vi "4. MassData in CSM.vi"() -> ()   [LabVIEW 2017]
doc: "## Using MassData in the CSM Framework (4. MassData in CSM.vi)\n\n### Overview\n\nDemonstrates how to use MassData within the CSM framework.\n\n### Introduction\n\nThis example uses a Producer/Consumer scenario to show how MassData operates within the CSM context.\n\nA non-CSM loop acts as the data producer, responsible for generating data, packing the data into a MassData argument, and sending the data via a synchronous message to the CSM module, which acts as the data consumer. This example demonstrates this process.\n\n### Steps\n\n- Step 1: Use `CSM - Config MassData Parameter Cache Size.vi` to set the cache size.\n- Step 2: Data producer loop. This loop is not a CSM module.\n - Step 2.1: Construct raw data, which in a real-world program comes from hardware acquisition, data reception, etc. Call `CSM - Convert MassData to Argument.vim` to convert the raw data into a MassData argument.\n - Step 2.2: Use `CSM - Wait and Send Message for Reply.vi` to send the data as an argument for `API: Update Waveform` to the CSM module, marking the sender as data producer.\n - Step 2.3: Data is sent only when the Generate button is pressed.\n - Step 2.4: (Optional) Use `CSM - MassData Update Status Indicator.vi` to update the cache status indicator on the UI.\n- Step 3: Data consumer loop. This loop is a CSM module named \"CSM\".\n - Step 3.1: In the `API: Update Waveform` case, take the received argument and use `CSM - Convert Argument to MassData.vim` to convert the MassData argument back to raw data and display the data.\n - Step 3.3: (Optional) Other cases remain consistent with the template and are unmodified.\n- Step 4: During the program exit process, use `CSM - Wait and Send Message for Reply.vi` to send the synchronous message \"Macro: Exit\" to the CSM module, causing the CSM module to shut down."
uses:
  addons/MassData-Parameter/Utility/Def-MassData Status Indicator(Vertical).ctl
  0ad19c59-6957-4552-8fdd-b1676ef9376a.vi
  2bb6a71f-0a6a-4702-91b6-10aea49c5400.vi
  28d1ee53-4aa5-43f0-882d-bc3139b7d369.vi
  d4bb06cd-b434-4495-85b0-046536fbf8bb.vi
  <userlib>/_NEVSTOP/Communicable State Machine(CSM)/AdvanceAPI/CSM - Revert Arguments-Safe String.vi
  <userlib>/_NEVSTOP/Communicable State Machine(CSM)/AdvanceAPI/CSM - Make String Arguments Safe.vi
  <userlib>/_NEVSTOP/Communicable State Machine(CSM)/AdvanceAPI/CSM - Break Down Multiple States String.vi
  <userlib>/_NEVSTOP/Communicable State Machine(CSM)/AdvanceAPI/CSM - Compact Multiple States.vi
  <userlib>/_NEVSTOP/Communicable State Machine(CSM)/AdvanceAPI/CSM - Keywords.vi
  <userlib>/_NEVSTOP/Communicable State Machine(CSM)/_Shared/Trim Single-line Text.vi
  addons/MassData-Parameter/_support/FGV-MassData(lvlibp).vi
  <userlib>/_NEVSTOP/Communicable State Machine(CSM)/Utility/CSM Data Type String.vi
  addons/MassData-Parameter/CSM MassData Parameter Support.lvlib
  <userlib>/_NEVSTOP/Communicable State Machine(CSM)/Communicable State Machine.lvlib
panel:
  out "Arguments":string
  in  "DataType":enum16{"DBL Array", "Waveform"}(ring)
  out "Waveform Graph":dbl[](graph)
  out "State History":string
  in  "Generate":bool
  out "MassData Status Vertical":T1={"w"={287840.0, 276144.0}, "r"={287840.0, 276144.0}} {"r" scale=1.0..20000000.0 scale format="%#_6p"; "w" scale=1.0..20000000.0 scale format="%#_6p"}
  in  "stop":bool
  # "#CSM-Example overview\n\nDemonstrates how to use MassData within the CSM framework."
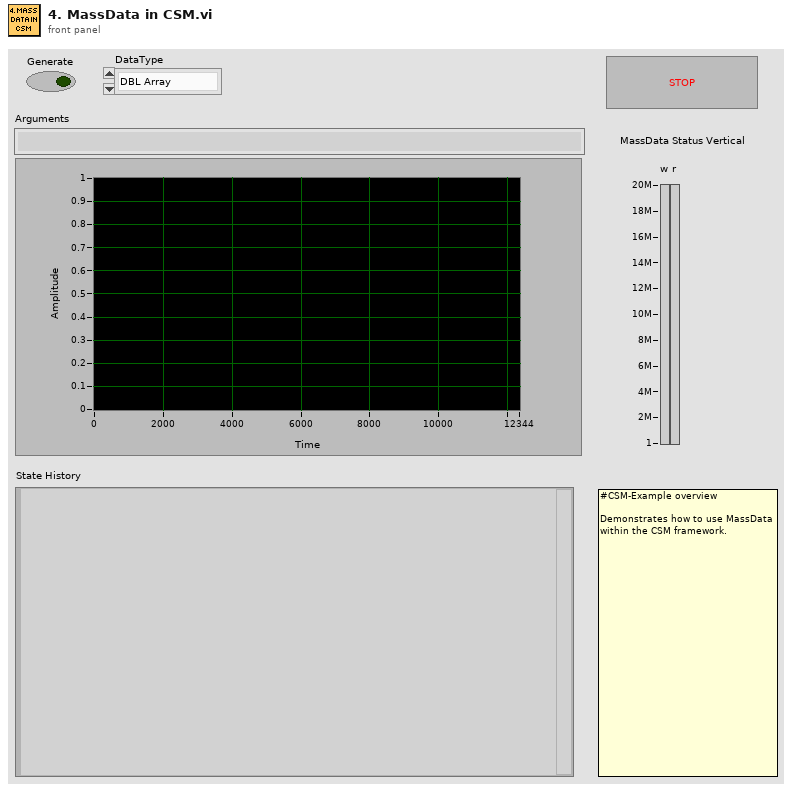
[diagram p1: front panel]
types:
  T1 = typedef "Def-MassData Status Indicator(Vertical).ctl" = cluster{"w":cluster{dbl, dbl}, "r":cluster{dbl, dbl}}
  T2 = enum32{"Invalid", "Standard", "Closed", "Hidden", "Minimized", "Maximized"}
  T3 = enum32{"invalid app kind", "Development System", "Run Time System", "Student Edition", "Embedded LabVIEW", "Evaluation", "Custom"}
  T4 = typedef "Communicable State Machine.lvlib/_CSM_Response Source Message.ctl" = cluster{"‘State":string, "’Arguments":string, "’Error":errorcluster}
  T5 = cluster{"Current VI Reference":refnum<vi>, "Close Panel on Exit?":bool}
  T6 = cluster{"Core":cluster{"Current VI Reference":refnum<vi>, "Close Panel on Exit?":bool}, "Your Boolean data":bool, "Your string data":string}
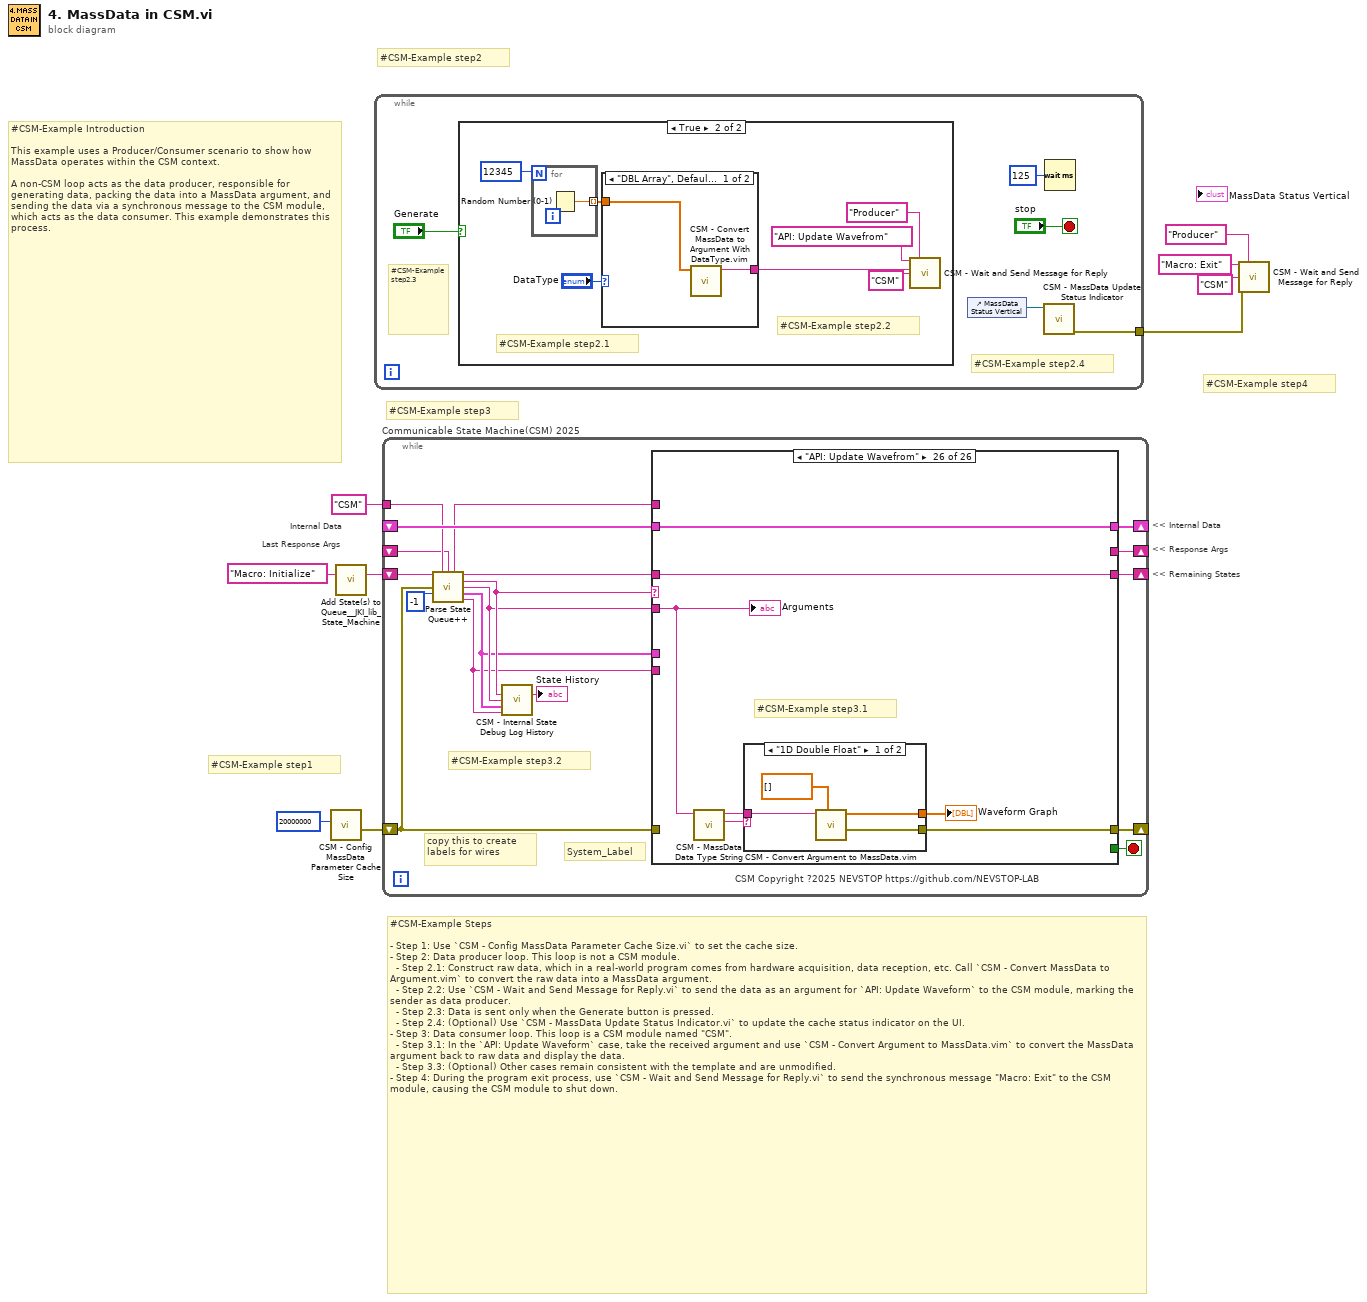
[diagram p0: block diagram]
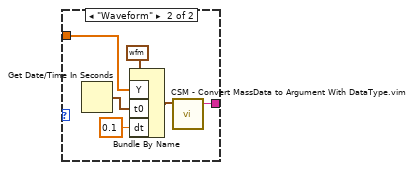
[diagram p3: hidden frame]
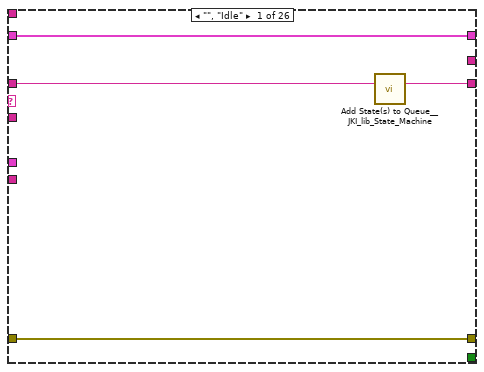
[diagram p4: hidden frame]
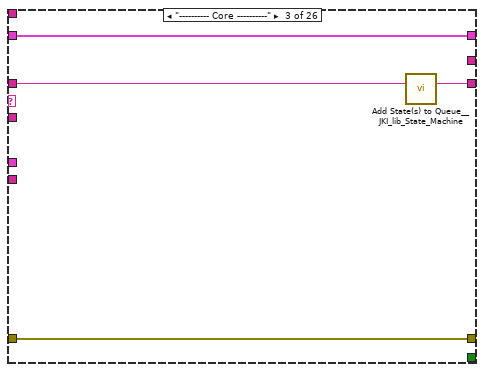
[diagram p6: hidden frame]
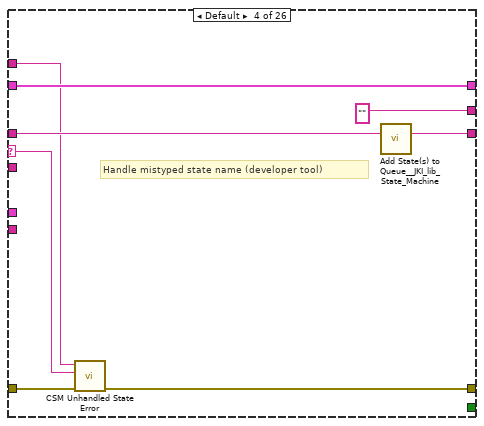
[diagram p7: hidden frame]
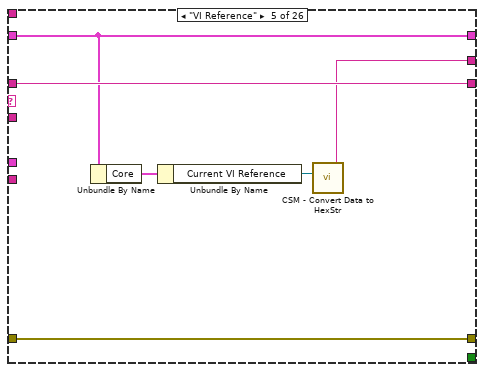
[diagram p8: hidden frame]
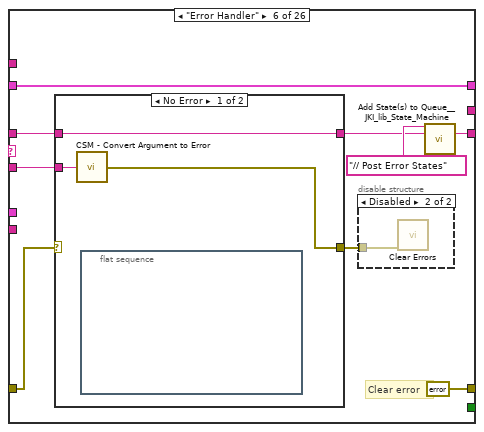
[diagram p9: hidden frame]
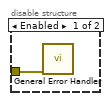
[diagram p10: hidden frame]
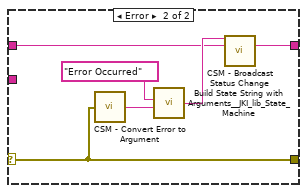
[diagram p11: hidden frame]
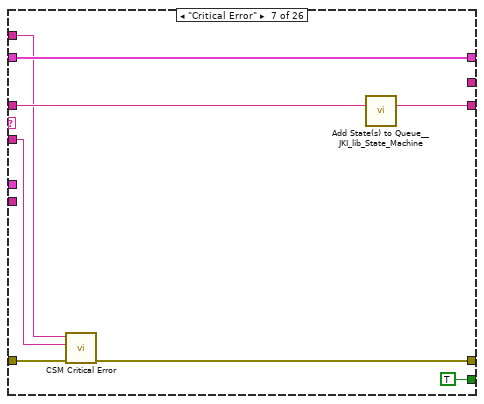
[diagram p12: hidden frame]
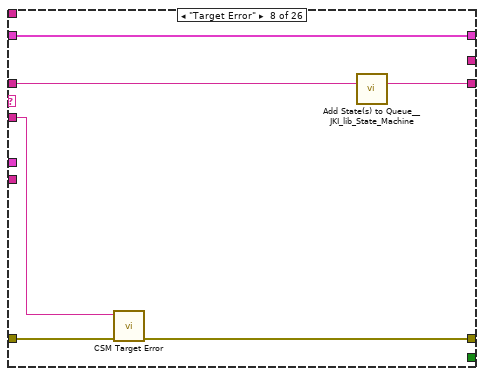
[diagram p13: hidden frame]
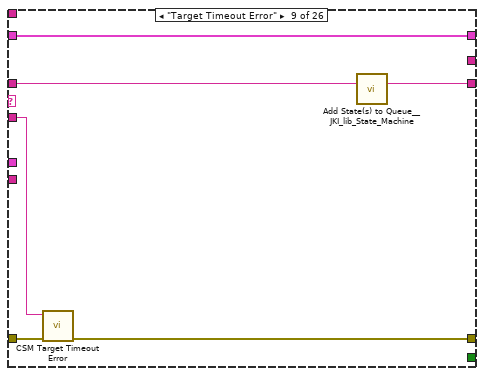
[diagram p14: hidden frame]
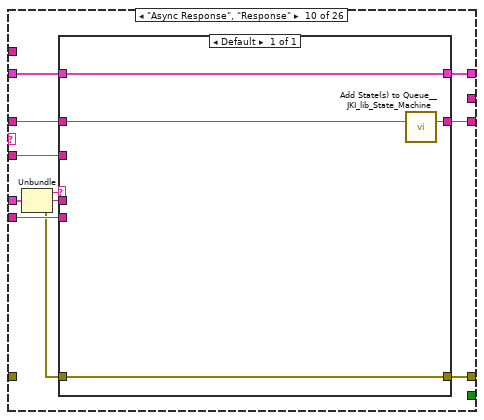
[diagram p15: hidden frame]
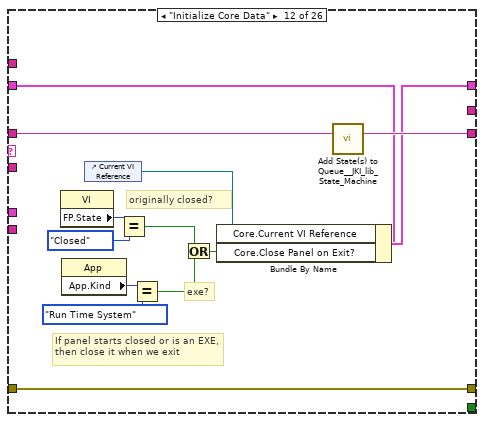
[diagram p17: hidden frame]
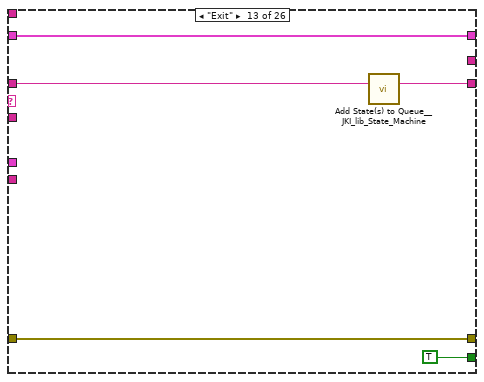
[diagram p18: hidden frame]
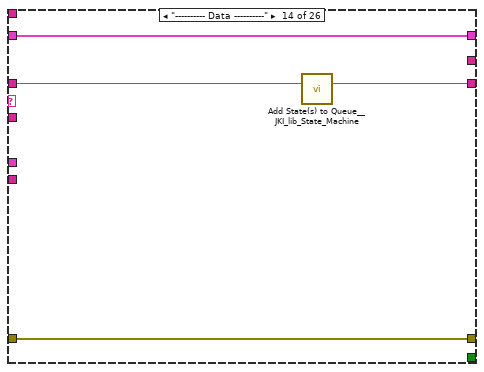
[diagram p19: hidden frame]
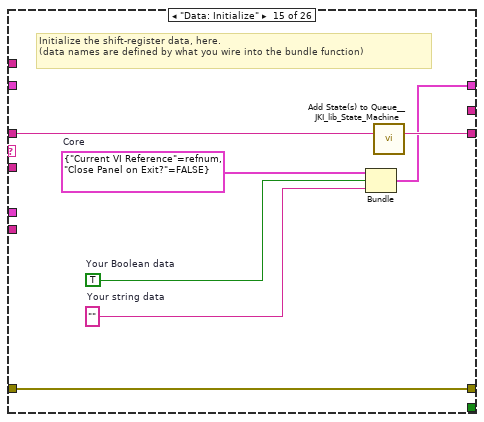
[diagram p20: hidden frame]
diagram:
  # "#CSM-Example step4"
  # "#CSM-Example step3"
  # "#CSM-Example step2"
  # "#CSM-Example step1"
  # "#CSM-Example Steps\n\n- Step 1: Use `CSM - Config MassData Parameter Cache Size.vi` to set the cache size.\n- Step 2: Data producer loop. This loop is not a CSM module.\n  - Step 2.1: Construct raw data, which in a real-world program comes from hardware acquisition, data reception, etc. Call `CSM - Convert MassData to Argument.vim` to convert the raw data into a MassData argument.\n  - Step 2.2: Use `CSM - Wait and Send Message for Reply.vi` to send the data as an argument for `API: Update Waveform` to the CSM module, marking the sender as data producer.\n  - Step 2.3: Data is sent only when the Generate button is pressed.\n  - Step 2.4: (Optional) Use `CSM - MassData Update Status Indicator.vi` to update the cache status indicator on the UI.\n- Step 3: Data consumer loop. This loop is a CSM module named \"CSM\".\n  - Step 3.1: In the `API: Update Waveform` case, take the received argument and use `CSM - Convert Argument to MassData.vim` to convert the MassData argument back to raw data and display the data.\n  - Step 3.3: (Optional) Other cases remain consistent with the template and are unmodified.\n- Step 4: During the program exit process, use `CSM - Wait and Send Message for Reply.vi` to send the synchronous message \"Macro: Exit\" to the CSM module, causing the CSM module to shut down."
  # "#CSM-Example Introduction\n\nThis example uses a Producer/Consumer scenario to show how MassData operates within the CSM context.\n\nA non-CSM loop acts as the data producer, responsible for generating data, packing the data into a MassData argument, and sending the data via a synchronous message to the CSM module, which acts as the data consumer. This example demonstrates this process."
  # "Last Response Args"
  # "Internal Data"
  # "<< Internal Data"
  # "<< Response Args"
  # "<< Remaining States"
  n1 = call "CSM - Config MassData Parameter Cache Size.vi"("Size (1M)"=20000000 ("size(1M)")) -> ("Error out"=w5:errorcluster)  [unwired: 10 in]
  n2 = call <vilib>:"Add State(s) to Queue__JKI_lib_State_Machine.vi"("State(s) in (\"\")"="Macro: Initialize" ("Init State(\"Macro: Initialize\")")) -> ("States Out"=w6:string)  [unwired: 14 in]
  n3 = while {
    tunnel: [w10] -> w3
    stop <- "stop" stop-if-true
    # "#CSM-Example step2.4"
    # "#CSM-Example step2.3"
    n4 = case shown="True" "Generate" {
      frame False {
      }
      frame True {
        # "#CSM-Example step2.2"
        # "#CSM-Example step2.1"
        n5 = for {
          N: 12345 -> [_]
          tunnel: [w30] -> w21 mode=indexing
          n6 = Random Number (0-1)() -> (number: 0 to 1=w30:dbl)
        }
        n7 = case shown="\"DBL Array\", Default" "DataType" {
          tunnel: w21 -> [w23 w29]
          tunnel: [w22 w25] -> w19
          frame "DBL Array", Default {
            n8 = call "CSM - Convert MassData to Argument With DataType.vim"("Data"=w23) -> ("MassData Argument"=w22:string)  [unwired: 7 in, 1 out]
          }
          frame "Waveform" {
            n9 = Get Date/Time In Seconds() -> (seconds since 1Jan1904=w28:timestamp)
            n10 = Bundle By Name(cluster=waveform(dbl) {"t0"=timestamp(0 s since 1904-01-01), "dt"=1.0, "Y"=[]} ("Waveform"), "Y"=w29, "t0"=w28, "dt"=0.1) -> (w24:waveform(dbl))
            n11 = call "CSM - Convert MassData to Argument With DataType.vim"("Data"=w24) -> ("MassData Argument"=w25:string)  [unwired: 7 in, 1 out]
          }
        }
        n12 = call <userlib>:"CSM - Wait and Send Message for Reply.vi"("State"="API: Update Wavefrom", "Current Module (\"\" to Generate an ID)"="Producer" ("Current Module(\"\" to generate a ID)"), "Arguments (\"\")"=w19, "Target Module"="CSM" ("Name(\"\" to use uuid)")) -> ()  [unwired: 9 in, 3 out]
      }
    }
    n13 = control-ref of="MassData Status Vertical"() -> (w11:refnum<vi>)
    n14 = call "CSM - MassData Update Status Indicator.vi"("MassData Status Indicator"=w11) -> ("error out"=w10:errorcluster)  [unwired: 10 in]
    n15 = Wait (ms)(milliseconds to wait=u32 125) -> ()  [unwired: 1 out]
  }
  n16 = while "Communicable State Machine(CSM) 2025" {
    shift-right: [w43] -> _
    shift-left: _ -> [w42]
    shift-right: [w46] -> _
    shift-left: w5 -> [w41]
    shift-right: [w45] -> _
    shift-left: w6 -> [w47]
    tunnel: "CSM" ("Name(\"\" to use uuid)") -> [w39]
    shift-right: [w40] -> _
    shift-left: _ -> [w33]
    stop <- w44 stop-if-true
    # "#CSM-Example step3.2"
    # "copy this to create labels for wires"
    # "System_Label"
    # "CSM Copyright ?2025 NEVSTOP https://github.com/NEVSTOP-LAB"
    n17 = call <userlib>:"Parse State Queue++.vi"("State Queue"=w47, "Name (\"\" to Use UUID)"=w39, "Response Arguments"=w33, "Previous Error"=w41, "Dequeue (1 ms)"=-1 ("Timeout")) -> ("Name Used"=w34:string, "Remaining States"=w48:string, "Current State"=w38:string, "Arguments"=w37:string, "Additional Information"=w36:T4, "Source CSM"=w35:string)  [unwired: 5 in]
    n18 = call <userlib>:"CSM - Internal State Debug Log History.vi"("State"=w38, "Arguments (\"\")"=w37, ">> Response Source Message >>"=w36, "Source (\"\")"=w35) -> ("Debug Log"=→"State History":string)  [unwired: 11 in]
    n19 = case shown="\"API: Update Wavefrom\"" w38 {
      selector: w38 -> [_ _ _ w62 _ _ _ _ _ _ _ _ _ _ _ _ _ _ _ _ _ _ _ _ _ _]
      tunnel: w48 -> [w49 w54 w59 w66 w72 w78 w99 w105 w111 w119 w130 w144 w149 w153 w160 w162 w169 w173 w177 w183 w198 w267 w272 w279 w281 w289]
      tunnel: w37 -> [_ _ _ _ _ w77 w95 w104 w109 w118 _ _ _ _ _ _ _ _ _ w178 w192 _ _ _ _ w285]
      tunnel: w42 -> [w50 w53 w56 w64 w71 w81 w100 w106 w112 w121 w129 w137 w147 w150 _ w161 w164 w170 w175 w181 w194 w264 w269 w276 w280 w288]
      tunnel: [w51 w55 w57 w60 w73 errorcluster {"status"=FALSE, "code"=0, "source"=""} ("error out") w96 w102 w108 w124 w131 w141 w146 w151 w157 w163 w165 w171 w174 w179 w195 w265 w270 w277 w282 w286] -> w46
      tunnel: w41 -> [w51 w55 w57 w67 w73 w79 w101 w103 w110 _ w131 w141 w146 w151 w157 w163 w166 w171 w174 w180 w196 w265 w270 w277 w282 _]
      tunnel: [w52 w54 w58 w65 w72 w74 w98 w107 w113 w120 w130 w143 w148 w152 w159 w162 w168 w172 w176 w182 w197 w266 w271 w278 w281 w289] -> w45
      tunnel: [_ _ _ _ _ _ TRUE _ _ _ _ _ TRUE _ _ _ _ _ _ _ _ _ _ _ _ _] -> w44
      tunnel: [w50 w53 w56 w64 w71 w81 w100 w106 w112 w122 w129 w142 w147 w150 w158 w161 w164 w170 w175 w181 w194 w264 w269 w276 w280 w288] -> w43
      tunnel: w35 -> [_ _ _ _ _ _ _ _ _ w116 _ _ _ _ _ _ _ _ _ _ _ _ _ _ _ _]
      tunnel: w36 -> [_ _ _ _ _ _ _ _ _ w123 _ _ _ _ _ _ _ _ _ _ _ _ _ _ _ _]
      tunnel: [_ _ _ "" w68 _ _ _ _ _ _ _ _ _ _ _ _ _ _ _ _ _ _ _ _ _] -> w40
      tunnel: w34 -> [_ _ _ w61 _ _ w94 _ _ _ _ _ _ _ _ _ _ _ _ _ _ _ _ _ _ _]
      frame "", "Idle" {
        n20 = call <vilib>:"Add State(s) to Queue__JKI_lib_State_Machine.vi"("State(s) in (\"\")"=w49) -> ("States Out"=w52:string)  [unwired: 14 in]
      }
      frame "CSM Documentation" {
      }
      frame "---------- Core ----------" {
        n21 = call <vilib>:"Add State(s) to Queue__JKI_lib_State_Machine.vi"("State(s) in (\"\")"=w59) -> ("States Out"=w58:string)  [unwired: 14 in]
      }
      frame Default {
        # "Handle mistyped state name (developer tool)"
        n22 = call <userlib>:"CSM Unhandled State Error.vi"("error in (no error)"=w67, "Undefined State"=w62, "CSM Name"=w61) -> ("error out"=w60:errorcluster)  [unwired: 8 in]
        n23 = call <vilib>:"Add State(s) to Queue__JKI_lib_State_Machine.vi"("State(s) in (\"\")"=w66) -> ("States Out"=w65:string)  [unwired: 14 in]
      }
      frame "VI Reference" {
        n24 = Unbundle By Name(w71) -> ("Core"=w70:T5)
        n25 = Unbundle By Name(w70) -> ("Current VI Reference"=w69:refnum<vi>)
        n26 = call <userlib>:"CSM - Convert Data to HexStr.vi"("Variant"=w69) -> ("HEX String (0-9,A-F)"=w68:string)  [unwired: 8 in]
      }
      frame "Error Handler" {
        # "Clear error"
        n27 = case shown="No Error" w79 {
          selector: w79 -> [_ w88]
          tunnel: [w87 w90] -> w75
          tunnel: w78 -> [w87 w89]
          tunnel: w77 -> [w86 _]
          tunnel: [w85 w88] -> w80
          frame No Error {
            n28 = call <userlib>:"CSM - Convert Argument to Error.vi"("Argument"=w86) -> ("Error"=w85:errorcluster)  [unwired: 4 in]
            n29 = flat-sequence {
              frame #0 {
              }
            }
          }
          frame Error {
            n30 = call <userlib>:"CSM - Convert Error to Argument.vi"("Error"=w88) -> ("Argument"=w92:string)  [unwired: 4 in]
            n31 = call <vilib>:"Build State String with Arguments__JKI_lib_State_Machine.vi"("Arguments (\"\")"=w92, "State"="Error Occurred" ("Status with Arguments")) -> ("State with Arguments"=w91:string)  [unwired: 4 in]
            n32 = call <userlib>:"CSM - Broadcast Status Change.vi"("Status With Arguments"=w91, "State Queue"=w89) -> ("Remaining States"=w90:string)  [unwired: 13 in]
          }
        }
        n33 = disable-structure shown="Disabled" {
          disable-tunnel: w80 -> [w83 w84]
          frame Enabled {
            n34 = call <vilib>:"General Error Handler.vi"("error in (no error)"=w83) -> ()  [unwired: 10 in, 5 out]
          }
          frame Disabled {
            n35 = call <vilib>:"Clear Errors.vi"("error in (no error)"=w84) -> ()  [unwired: 5 in, 2 out]
          }
        }
        n36 = call <vilib>:"Add State(s) to Queue__JKI_lib_State_Machine.vi"("State(s) in Front (\"\")"="// Post Error States", "State(s) in (\"\")"=w75) -> ("States Out"=w74:string)  [unwired: 13 in]
      }
      frame "Critical Error" {
        n37 = call <userlib>:"CSM Critical Error.vi"("error in (no error)"=w101, "Arugments (As Reason)"=w95, "CSM Name"=w94) -> ("error out"=w96:errorcluster)  [unwired: 8 in]
        n38 = call <vilib>:"Add State(s) to Queue__JKI_lib_State_Machine.vi"("State(s) in (\"\")"=w99) -> ("States Out"=w98:string)  [unwired: 14 in]
      }
      frame "Target Error" {
        n39 = call <userlib>:"CSM Target Error.vi"("error in (no error)"=w103, "Arguments (As CSM Name)"=w104) -> ("error out"=w102:errorcluster)  [unwired: 9 in]
        n40 = call <vilib>:"Add State(s) to Queue__JKI_lib_State_Machine.vi"("State(s) in (\"\")"=w105) -> ("States Out"=w107:string)  [unwired: 14 in]
      }
      frame "Target Timeout Error" {
        n41 = call <userlib>:"CSM Target Timeout Error.vi"("error in (no error)"=w110, "Arguments (As CSM Name)"=w109) -> ("error out"=w108:errorcluster)  [unwired: 9 in]
        n42 = call <vilib>:"Add State(s) to Queue__JKI_lib_State_Machine.vi"("State(s) in (\"\")"=w111) -> ("States Out"=w113:string)  [unwired: 14 in]
      }
      frame "Async Response", "Response" {
        n43 = Unbundle(w123) -> ("‘State"=w117:string, "’Arguments"=w115:string, "’Error"=w114:errorcluster)
        n44 = case shown="Default" w117 {
          tunnel: [w128] -> w124
          tunnel: w114 -> [w128]
          tunnel: [w127] -> w122
          tunnel: w121 -> [w127]
          tunnel: [w125] -> w120
          tunnel: w119 -> [w126]
          tunnel: w118 -> [_]
          tunnel: w116 -> [_]
          tunnel: w115 -> [_]
          frame Default {
            n45 = call <vilib>:"Add State(s) to Queue__JKI_lib_State_Machine.vi"("State(s) in (\"\")"=w126) -> ("States Out"=w125:string)  [unwired: 14 in]
          }
        }
      }
      frame "Async Message Posted" {
      }
      frame "Initialize Core Data" {
        # "originally closed?"
        # "exe?"
        # "If panel starts closed or is an EXE, then close it when we exit"
        n46 = property class="VI"() -> ("FP.State"=w134:T2)  [unwired: 2 in, 2 out]
        n47 = property class="App"() -> ("App.Kind"=w140:T3)  [unwired: 2 in, 2 out]
        n48 = control-ref of="Current VI Reference"() -> (w135:refnum<vi>)
        n49 = Equal?(x=w134, y=T2."Closed" ("Front Panel Window:State")) -> (x = y?=w132:bool)
        n50 = Equal?(x=w140, y=T3."Run Time System" ("Application:Kind")) -> (x = y?=w138:bool)
        n51 = Or(x=w132, y=w138) -> (x .or. y?=w136:bool)
        n52 = Bundle By Name(cluster=w137, "Core.Current VI Reference"=w135, "Core.Close Panel on Exit?"=w136) -> (w142:T6)
        n53 = call <vilib>:"Add State(s) to Queue__JKI_lib_State_Machine.vi"("State(s) in (\"\")"=w144) -> ("States Out"=w143:string)  [unwired: 14 in]
      }
      frame "Exit" {
        n54 = call <vilib>:"Add State(s) to Queue__JKI_lib_State_Machine.vi"("State(s) in (\"\")"=w149) -> ("States Out"=w148:string)  [unwired: 14 in]
      }
      frame "---------- Data ----------" {
        n55 = call <vilib>:"Add State(s) to Queue__JKI_lib_State_Machine.vi"("State(s) in (\"\")"=w153) -> ("States Out"=w152:string)  [unwired: 14 in]
      }
      frame "Data: Initialize" {
        w154 = T5 {"Current VI Reference"=refnum, "Close Panel on Exit?"=FALSE}  # Core
        w156 = TRUE  # Your Boolean data
        w155 = ""  # Your string data
        # "Initialize the shift-register data, here.\n(data names are defined by what you wire into the bundle function)"
        n56 = Bundle("Core"=w154, "Your Boolean data"=w156, "Your string data"=w155) -> (w158:T6)  [unwired: 1 in]
        n57 = call <vilib>:"Add State(s) to Queue__JKI_lib_State_Machine.vi"("State(s) in (\"\")"=w160) -> ("States Out"=w159:string)  [unwired: 14 in]
      }
      frame "Data: Update Indicators" {
      }
      frame "Data: Cleanup" {
        # "Cleanup any data and references, here.\n(this is called automatically, by the Macro: Exit)"
        n58 = Unbundle By Name(w164) -> ("Core.Current VI Reference"=w167:refnum<vi>)
        n59 = Close Reference(reference=w167, error in (no error)=w166) -> (error out=w165:errorcluster)
        n60 = call <vilib>:"Add State(s) to Queue__JKI_lib_State_Machine.vi"("State(s) in (\"\")"=w169) -> ("States Out"=w168:string)  [unwired: 14 in]
      }
      frame "---------- UI ----------" {
        n61 = call <vilib>:"Add State(s) to Queue__JKI_lib_State_Machine.vi"("State(s) in (\"\")"=w173) -> ("States Out"=w172:string)  [unwired: 14 in]
      }
      frame "UI: Initialize" {
        n62 = call <vilib>:"Add State(s) to Queue__JKI_lib_State_Machine.vi"("State(s) in (\"\")"=w177) -> ("States Out"=w176:string)  [unwired: 14 in]
      }
      frame "UI: Cursor Set" {
        # "Argument"
        n63 = disable-structure shown="TARGET_TYPE!=Windows" {
          disable-tunnel: w180 -> [w186 w191]
          disable-tunnel: [w185 w191] -> w179
          disable-tunnel: w178 -> [w184 _]
          frame condition #0 (active) {
            n64 = case shown="\"Idle\", Default" w184 {
              tunnel: w186 -> [w188 w190]
              tunnel: [w187 w189] -> w185
              frame "Idle", Default {
                n65 = call <vilib>:"Unset Busy.vi"("error in (no error)"=w188) -> ("error out"=w187:errorcluster)  [unwired: 10 in]
              }
              frame "Busy" {
                n66 = call <vilib>:"Set Busy.vi"("error in (no error)"=w190) -> ("error out"=w189:errorcluster)  [unwired: 9 in, 1 out]
              }
            }
          }
          frame condition #1 {
          }
        }
        n67 = call <vilib>:"Add State(s) to Queue__JKI_lib_State_Machine.vi"("State(s) in (\"\")"=w183) -> ("States Out"=w182:string)  [unwired: 14 in]
      }
      frame "UI: Front Panel State" {
        # "Argument"
        n68 = Unbundle By Name(w194) -> ("Core.Current VI Reference"=w193:refnum<vi>)
        n69 = call <vilib>:"Add State(s) to Queue__JKI_lib_State_Machine.vi"("State(s) in (\"\")"=w198) -> ("States Out"=w197:string)  [unwired: 14 in]
        n70 = case shown="\"Close\", \"Closed\"" w192 {
          tunnel: w196 -> [w204 w219 w230 w243 w256]
          tunnel: [w206 w220 w232 w245 w258] -> w195
          tunnel: w193 -> [w205 w217 w231 w244 w257]
          frame "Open", "Standard", Default {
            w199 = T2."Standard" ("State")
            n71 = property class="VI"(reference=w205, error in=w204) -> (reference out=w202:refnum<vi>, error out=w203:errorcluster, "FP.State"=w201:T2)
            n72 = Not Equal?(x=w201, y=w199) -> (x != y?=w200:bool)
            n73 = case shown="True" w200 {
              tunnel: [w210 w212] -> w206
              tunnel: w203 -> [w209 w212]
              tunnel: w202 -> [w208 _]
              tunnel: w199 -> [w207 _]
              frame True {
                n74 = invoke class="VI" method="FP.Open"(reference=w208, error in=w209, "Activate"=TRUE, "State"=w207) -> (error out=w210:errorcluster)  [unwired: 1 in, 4 out]
              }
              frame False {
              }
            }
          }
          frame "Close", "Closed" {
            n75 = property class="VI"(reference=w217, error in=w219) -> (reference out=w216:refnum<vi>, error out=w218:errorcluster, "FP.State"=w214:T2)
            n76 = Not Equal?(x=w214, y=T2."Closed" ("Front Panel Window:State")) -> (x != y?=w213:bool)
            n77 = case shown="False" w213 {
              tunnel: [w221 w224] -> w220
              tunnel: w218 -> [w221 w223]
              tunnel: w216 -> [_ w222]
              frame False {
              }
              frame True {
                n78 = invoke class="VI" method="FP.Close"(reference=w222, error in=w223) -> (error out=w224:errorcluster)  [unwired: 1 in, 2 out]
              }
            }
          }
          frame "Hidden", "Hide" {
            w225 = T2."Hidden" ("State")
            n79 = property class="VI"(reference=w231, error in=w230) -> (reference out=w228:refnum<vi>, error out=w229:errorcluster, "FP.State"=w227:T2)
            n80 = Not Equal?(x=w227, y=w225) -> (x != y?=w226:bool)
            n81 = case shown="True" w226 {
              tunnel: [w236 w237] -> w232
              tunnel: w229 -> [w235 w237]
              tunnel: w228 -> [w234 _]
              tunnel: w225 -> [w233 _]
              frame True {
                n82 = invoke class="VI" method="FP.Open"(reference=w234, error in=w235, "State"=w233) -> (error out=w236:errorcluster)  [unwired: 2 in, 4 out]
              }
              frame False {
              }
            }
          }
          frame "Minimize", "Minimized" {
            w238 = T2."Minimized" ("State")
            n83 = property class="VI"(reference=w244, error in=w243) -> (reference out=w241:refnum<vi>, error out=w242:errorcluster, "FP.State"=w240:T2)
            n84 = Not Equal?(x=w240, y=w238) -> (x != y?=w239:bool)
            n85 = case shown="True" w239 {
              tunnel: [w249 w250] -> w245
              tunnel: w242 -> [w248 w250]
              tunnel: w241 -> [w247 _]
              tunnel: w238 -> [w246 _]
              frame True {
                n86 = invoke class="VI" method="FP.Open"(reference=w247, error in=w248, "State"=w246) -> (error out=w249:errorcluster)  [unwired: 2 in, 4 out]
              }
              frame False {
              }
            }
          }
          frame "Maximize", "Maximized" {
            w251 = T2."Maximized" ("State")
            n87 = property class="VI"(reference=w257, error in=w256) -> (reference out=w254:refnum<vi>, error out=w255:errorcluster, "FP.State"=w253:T2)
            n88 = Not Equal?(x=w253, y=w251) -> (x != y?=w252:bool)
            n89 = case shown="True" w252 {
              tunnel: [w262 w263] -> w258
              tunnel: w255 -> [w261 w263]
              tunnel: w254 -> [w260 _]
              tunnel: w251 -> [w259 _]
              frame True {
                n90 = invoke class="VI" method="FP.Open"(reference=w260, error in=w261, "State"=w259) -> (error out=w262:errorcluster)  [unwired: 2 in, 4 out]
              }
              frame False {
              }
            }
          }
        }
      }
      frame "---------- Macro ----------" {
        n91 = call <vilib>:"Add State(s) to Queue__JKI_lib_State_Machine.vi"("State(s) in (\"\")"=w267) -> ("States Out"=w266:string)  [unwired: 14 in]
      }
      frame "Macro: Initialize" {
        n92 = call <vilib>:"Add State(s) to Queue__JKI_lib_State_Machine.vi"("State(s) in Front (\"\")"="Data: Initialize\nInitialize Core Data\nData: Update Indicators", "State(s) in (\"\")"=w272) -> ("States Out"=w271:string)  [unwired: 13 in]
      }
      frame "Macro: Exit" {
        n93 = call <vilib>:"Add State(s) to Queue__JKI_lib_State_Machine.vi"("State(s) in Front (\"\")"="//Exit Sub-Modules ", "State(s) at Back (\"\")"="Data: Cleanup\nExit") -> ("States Out"=w274:string)  [unwired: 13 in]
        n94 = call <vilib>:"Add State(s) to Queue__JKI_lib_State_Machine.vi"("State(s) in Front (\"\")"=w274, "State(s) in (\"\")"=w279) -> ("States Out"=w278:string)  [unwired: 13 in]
      }
      frame "---------- API ----------" {
      }
      frame "API: Update Wavefrom" {
        # "#CSM-Example step3.1"
        n95 = call "CSM - MassData Data Type String.vi"("MassData Argument"=w285) -> ("Data Type String"=w283:string, "MassData Argument (dup)"=w284:string)  [unwired: 6 in, 1 out]
        n96 = case shown="\"1D Double Float\"" w283 {
          tunnel: [w291 w294] -> w287
          tunnel: [w290 w296] -> w286
          tunnel: w284 -> [w293 w295]
          frame "1D Double Float" {
            n97 = call "CSM - Convert Argument to MassData.vim"("Type"=dbl[] [], "MassData Argument"=w293) -> ("error out"=w290:errorcluster, "Data"=w291:dbl[])  [unwired: 6 in]
          }
          frame "Waveform", Default {
            n98 = call "CSM - Convert Argument to MassData.vim"("Type"=waveform(dbl) {"t0"=timestamp(0 s since 1904-01-01), "dt"=1.0, "Y"=[]} ("output waveform"), "MassData Argument"=w295) -> ("error out"=w296:errorcluster, "Data"=w297:waveform(dbl))  [unwired: 6 in]
            n99 = Unbundle By Name(w297) -> ("Y"=w294:dbl[])
          }
        }
        "Waveform Graph" <- w287
        "Arguments" <- w285
      }
    }
  }
  n100 = call <userlib>:"CSM - Wait and Send Message for Reply.vi"("State"="Macro: Exit", "Current Module (\"\" to Generate an ID)"="Producer" ("Current Module(\"\" to generate a ID)"), "Target Module"="CSM" ("Name(\"\" to use uuid)"), "Error In (No Error)"=w3) -> ()  [unwired: 9 in, 3 out]
